vi "AI Check For Empty Channels.vi"(1 "AI Configuration In":T1(array[cluster])=[{"AI.Coupling"=10050, "AI.Max"=10.0, "AI.Min"=-10.0, "Input physical channels"="PXI1Slot2/ai0:1"}, {"AI.Coupling"=10050, "AI.Max"=10.0, "AI.Min"=-10.0, "Input physical channels"="PXI1Slot3/ai0:1"}, {"AI.Coupling"=10050, "AI.Max"=10.0, "AI.Min"=-10.0, "Input physical channels"="PXI1Slot6/ai0:1"}] {"AI.Coupling" items=["AC"=10045, "DC"=10050, "GND"=10066]}) -> (0 "AI Configuration Out":T1(array[cluster]))   [LabVIEW 2013, in "Lock-In Variable Channels_2.lvclass"]
uses:
  Lock-In Variable Channels_2.lvclass
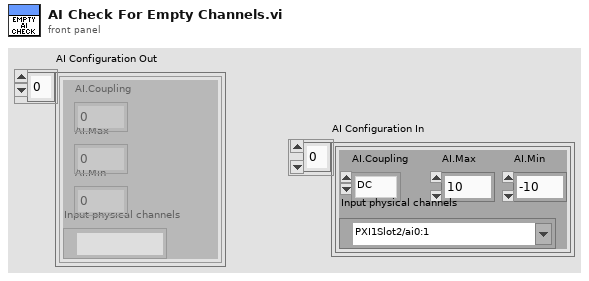
[diagram p1: front panel]
types:
  T1 = cluster{"AI.Coupling":i32, "AI.Max":dbl, "AI.Min":dbl, "Input physical channels":tag}[]
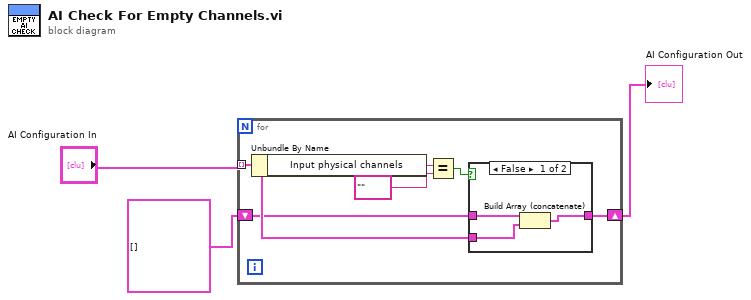
[diagram p0: block diagram]
diagram:
  n1 = for {
    tunnel: "AI Configuration In" -> [w6] mode=indexing
    shift-right: [w4] -> w3
    shift-left: T1 [] ("AI Configuration") -> [w5]
    n2 = Unbundle By Name(w6) -> ("Input physical channels"=w8:tag)
    n3 = Equal?(x=w8, y=tag "" ("Empty physical channels")) -> (x = y?=w9:bool)
    n4 = case shown="False" w9 {
      tunnel: w6 -> [w11 _]
      tunnel: w5 -> [w12 w13]
      tunnel: [w10 w13] -> w4
      frame False {
        n5 = Build Array (concatenate)(w12, w11) -> (w10:T1)
      }
      frame True {
      }
    }
  }
  "AI Configuration Out" <- w3
